vi "ExternalIN.vi"(0 "nDeviceNo":u32, 1 "Mode":u16(ring) items=["Get&Set", "Get", "Set"], 5 "nChildNo":u32, 9 "NewExternalInMode":u32[](array[numeric]), 11 "Error_In":T1) -> (3 "ExternalIn1ModeList":cluster{string, i32}[](array[cluster]), 4 "Error?":bool, 6 "ExternalIn1Mode":u32, 8 "ExternalIn2Mode":u32, 10 "ExternalIn3Mode":u32, 12 "ExternalIn2ModeList":cluster{string, i32}[](array[cluster]), 14 "ExternalIn3ModeList":cluster{string, i32}[](array[cluster]), 15 "Error_Out":T1)   [LabVIEW 2015]
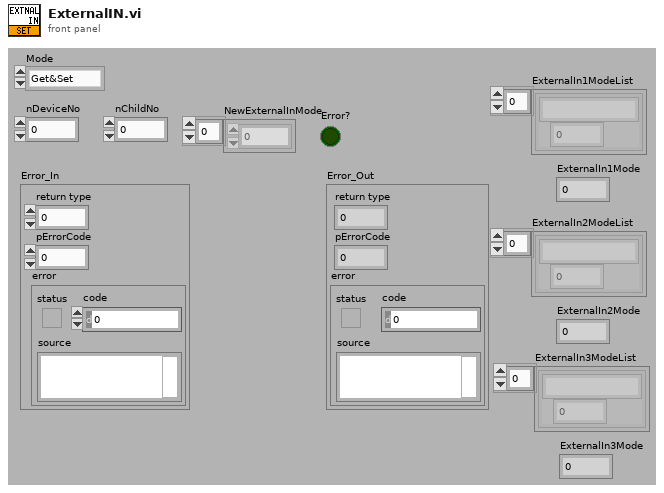
[diagram p1: front panel]
types:
  T1 = cluster{"return type":u32, "pErrorCode":u32, "error ":errorcluster}
  T2 = cluster{"ReturnValue":u32, "ErrorCode":u32, "error ":errorcluster}
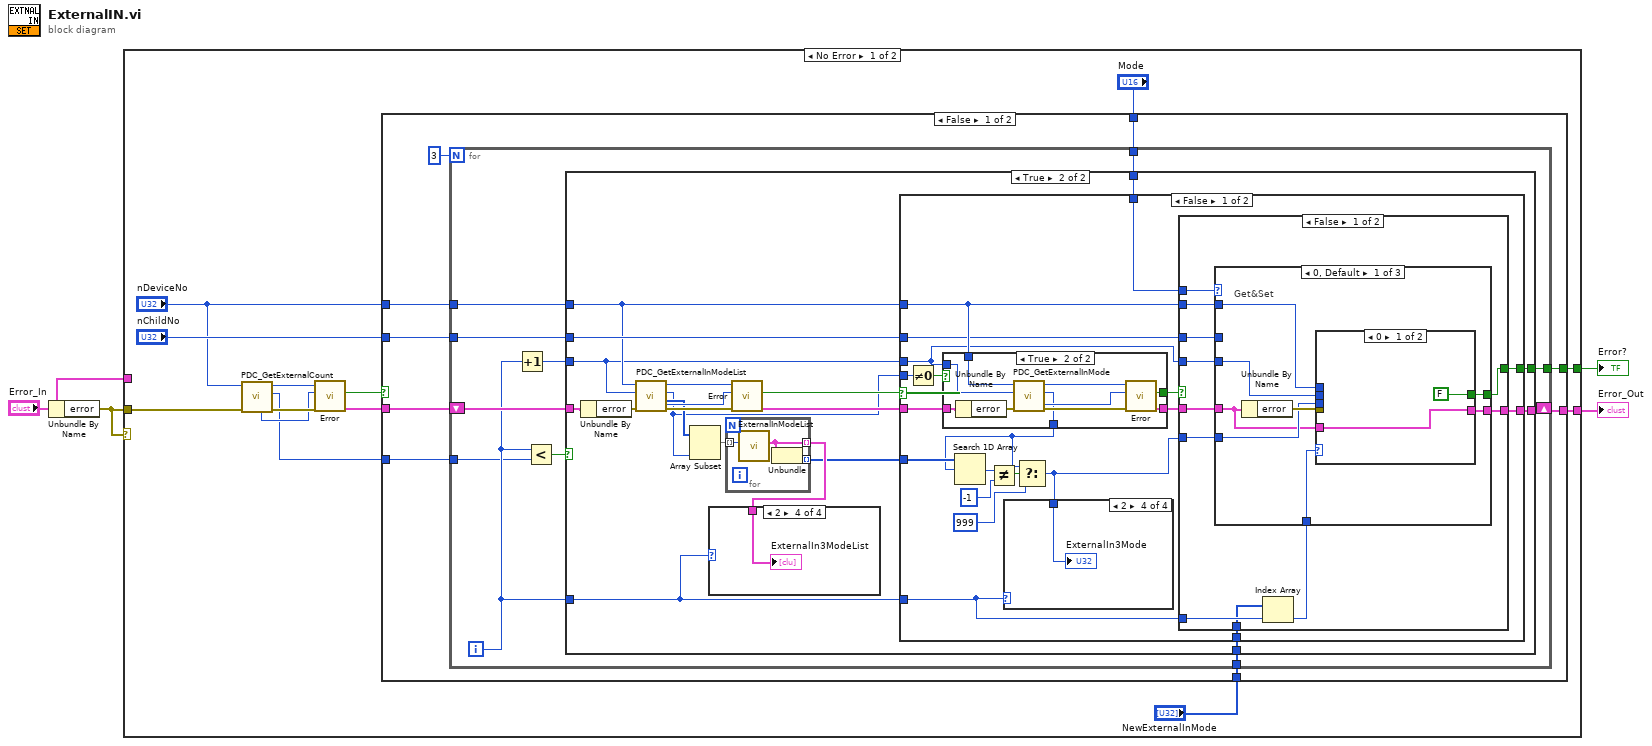
[diagram p0: block diagram]
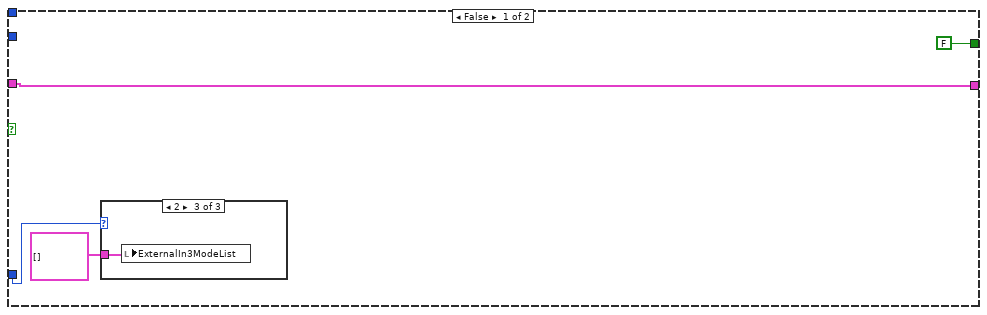
[diagram p2: hidden frame]
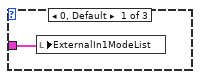
[diagram p3: hidden frame]
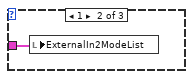
[diagram p4: hidden frame]
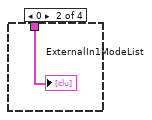
[diagram p6: hidden frame]
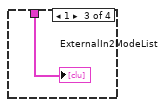
[diagram p7: hidden frame]
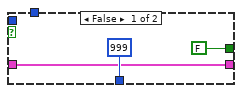
[diagram p8: hidden frame]
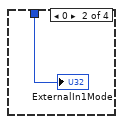
[diagram p10: hidden frame]
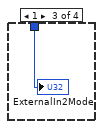
[diagram p11: hidden frame]
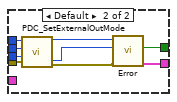
[diagram p12: hidden frame]
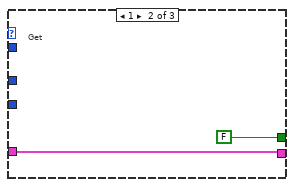
[diagram p13: hidden frame]
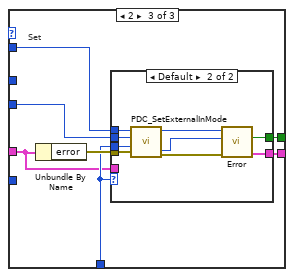
[diagram p14: hidden frame]
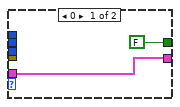
[diagram p15: hidden frame]
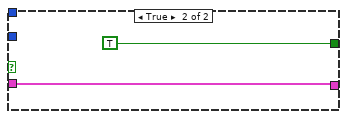
[diagram p16: hidden frame]
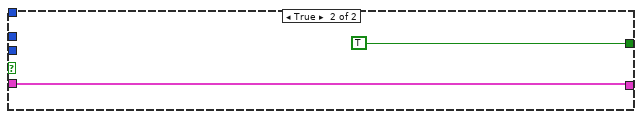
[diagram p17: hidden frame]
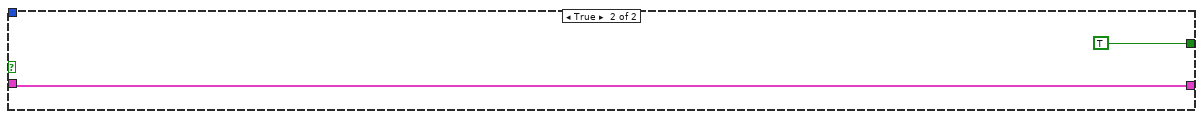
[diagram p18: hidden frame]
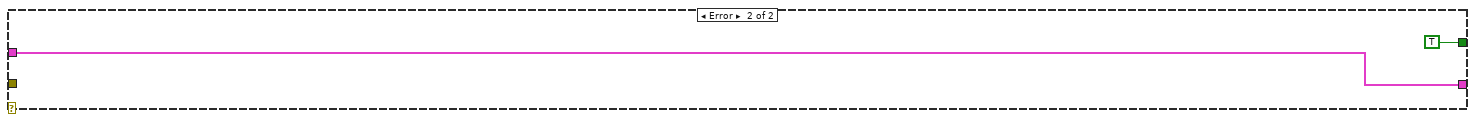
[diagram p19: hidden frame]
diagram:
  n1 = Unbundle By Name("Error_In") -> ("error"=w2:errorcluster)
  n2 = case shown="No Error" w2 {
    tunnel: [w17 w164] -> w4
    tunnel: [w16 TRUE ("Error?")] -> w3
    tunnel: w2 -> [w9 _]
    tunnel: "Error_In" -> [_ w164]
    frame No Error {
      n3 = call "PDC_GetExternalCount.vi"("error in (no error)"=w9, "DeviceNo"="nDeviceNo") -> ("error out"=w10:errorcluster, "In"=w5:u32, "ReturnValue"=w6:u32, "ErrorCode"=w7:u32)  [unwired: 6 out]
      n4 = call "Error.vi"("error in (no error)"=w10, "ErrorCode"=w7, "ReturnValue"=w6) -> ("Error_Out"=w12:T2, "Error?"=w13:bool)  [unwired: 7 out]
      n5 = case shown="False" w13 {
        tunnel: [w26 w161] -> w17
        tunnel: [w25 TRUE ("Error?")] -> w16
        tunnel: "nChildNo" -> [w24 _]
        tunnel: "nDeviceNo" -> [w23 _]
        tunnel: "Mode" -> [w22 _]
        tunnel: w12 -> [w21 w161]
        tunnel: "NewExternalInMode" -> [w20 _]
        tunnel: w5 -> [w18 _]
        frame False {
          n6 = for {
            N: 3 -> [_]
            tunnel: [w36] -> w25
            tunnel: w24 -> [w35]
            tunnel: w23 -> [w34]
            tunnel: w22 -> [w33]
            shift-right: [w37] -> w26
            shift-left: w21 -> [w32]
            tunnel: w20 -> [w31]
            tunnel: w18 -> [w27]
            i -> [w28]
            n7 = Increment(x=w28) -> (x+1=w30:i32)
            n8 = Less?(x=w28, y=w27) -> (x < y?=w29:bool)
            n9 = case shown="True" w29 {
              tunnel: [w41 w64] -> w37
              tunnel: [FALSE ("Error?") w63] -> w36
              tunnel: w35 -> [_ w62]
              tunnel: w34 -> [_ w55]
              tunnel: w33 -> [_ w53]
              tunnel: w32 -> [w41 w52]
              tunnel: w28 -> [w39 w50]
              tunnel: w30 -> [_ w49]
              tunnel: w31 -> [_ w48]
              frame False {
                n10 = case shown="2" w39 {
                  tunnel: cluster{string, i32}[] [] ("External\nGeneralOutModeList") -> [w42 w43 w44]
                  frame 0, Default {
                    n11 = local write "ExternalIn1ModeList"(w42) -> ()
                  }
                  frame 1 {
                    n12 = local write "ExternalIn2ModeList"(w43) -> ()
                  }
                  frame 2 {
                    n13 = local write "ExternalIn3ModeList"(w44) -> ()
                  }
                }
              }
              frame True {
                n14 = Unbundle By Name(w52) -> ("error"=w51:errorcluster)
                n15 = call "PDC_GetExternalInModeList.vi"("error in (no error)"=w51, "PortNo"=w49, "DeviceNo"=w55) -> ("error out"=w61:errorcluster, "List"=w57:u32[], "Size"=w45:u32, "ReturnValue"=w60:u32, "ErrorCode"=w59:u32)  [unwired: 4 out]
                n16 = Array Subset(array=w57, length=w45) -> (w58:u32[])  [unwired: 1 in]
                n17 = for {
                  tunnel: w58 -> [w160] mode=indexing
                  tunnel: [w159] -> w47 mode=indexing
                  tunnel: [w158] -> w46 mode=indexing
                  n18 = call "ExternalInModeList.vi"("List"=w160) -> ("GetLUTModeList"=w159:cluster{string, i32})  [unwired: 10 out]
                  n19 = Unbundle(w159) -> (w158:i32)  [unwired: 1 out]
                }
                n20 = case shown="2" w50 {
                  tunnel: w47 -> [_ w65 w66 w67]
                  frame Default {
                  }
                  frame 0 {
                    "ExternalIn1ModeList" <- w65
                  }
                  frame 1 {
                    "ExternalIn2ModeList" <- w66
                  }
                  frame 2 {
                    "ExternalIn3ModeList" <- w67
                  }
                }
                n21 = call "Error.vi"("error in (no error)"=w61, "ErrorCode"=w59, "ReturnValue"=w60) -> ("Error_Out"=w56:T2, "Error?"=w54:bool)  [unwired: 7 out]
                n22 = case shown="False" w54 {
                  tunnel: [w85 w157] -> w64
                  tunnel: [w84 TRUE ("Error?")] -> w63
                  tunnel: w56 -> [w83 w157]
                  tunnel: w55 -> [w82 _]
                  tunnel: w62 -> [w81 _]
                  tunnel: w49 -> [w70 _]
                  tunnel: w53 -> [w80 _]
                  tunnel: w50 -> [w79 _]
                  tunnel: w48 -> [w78 _]
                  tunnel: w46 -> [w77 _]
                  tunnel: w45 -> [w68 _]
                  frame False {
                    n23 = Not Equal To 0?(x=w68) -> (x != 0?=w69:bool)
                    n24 = case shown="True" w69 {
                      tunnel: [FALSE ("Error?") w97] -> w87
                      tunnel: [w89 w96] -> w86
                      tunnel: w83 -> [w89 w94]
                      tunnel: w82 -> [_ w93]
                      tunnel: w70 -> [_ w92]
                      tunnel: [u32 999 ("pMode") w91] -> w74
                      frame False {
                      }
                      frame True {
                        n25 = Unbundle By Name(w94) -> ("error"=w95:errorcluster)
                        n26 = call "PDC_GetExternalInMode.vi"("error in (no error)"=w95, "Port"=w92, "DeviceNo"=w93) -> ("error out"=w98:errorcluster, "Mode"=w91:u32, "ReturnValue"=w99:u32, "ErrorCode"=w100:u32)  [unwired: 5 out]
                        n27 = call "Error.vi"("error in (no error)"=w98, "ErrorCode"=w100, "ReturnValue"=w99) -> ("Error_Out"=w96:T2, "Error?"=w97:bool)  [unwired: 7 out]
                      }
                    }
                    n28 = Search 1D Array(1D array=w77, element=w74) -> (index of element=w76:i32)  [unwired: 1 out]
                    n29 = Not Equal?(x=w76, y=-1) -> (x != y?=w73:bool)
                    n30 = Select(t=w74, s=w73, f=u32 999 ("y")) -> (s? t:f=w72:u32)
                    n31 = case shown="2" w79 {
                      tunnel: w72 -> [_ w101 w102 w103]
                      frame Default {
                      }
                      frame 0 {
                        "ExternalIn1Mode" <- w101
                      }
                      frame 1 {
                        "ExternalIn2Mode" <- w102
                      }
                      frame 2 {
                        "ExternalIn3Mode" <- w103
                      }
                    }
                    n32 = case shown="False" w87 {
                      tunnel: w86 -> [w108 w155]
                      tunnel: [w114 w155] -> w85
                      tunnel: w82 -> [w111 _]
                      tunnel: w81 -> [w110 _]
                      tunnel: [w113 TRUE ("Error?")] -> w84
                      tunnel: w80 -> [w112 _]
                      tunnel: w72 -> [w109 _]
                      tunnel: w70 -> [w107 _]
                      tunnel: w79 -> [w106 _]
                      tunnel: w78 -> [w105 _]
                      frame False {
                        n33 = Index Array(array=w105, index=w106) -> (element=w104:u32)
                        n34 = case shown="0, Default" w112 {
                          tunnel: w108 -> [w115 w135 w136]
                          tunnel: [w121 w135 w141] -> w114
                          tunnel: w111 -> [w120 _ w140]
                          tunnel: w110 -> [_ _ _]
                          tunnel: [w119 FALSE ("Error?") w139] -> w113
                          tunnel: w109 -> [w118 _ _]
                          tunnel: w107 -> [w117 _ w138]
                          tunnel: w104 -> [w116 _ w137]
                          frame 0, Default {
                            # "Get&Set"
                            n35 = Unbundle By Name(w115) -> ("error"=w122:errorcluster)
                            n36 = case shown="0" w116 {
                              tunnel: w122 -> [_ w133]
                              tunnel: [w123 w129] -> w121
                              tunnel: w120 -> [_ w128]
                              tunnel: [FALSE ("Error?") w127] -> w119
                              tunnel: w118 -> [_ w126]
                              tunnel: w117 -> [_ w125]
                              tunnel: w115 -> [w123 _]
                              frame 0 {
                              }
                              frame Default {
                                n37 = call "PDC_SetExternalOutMode.vi"("error in (no error)"=w133, "Mode"=w126, "Port"=w125, "DeviceNo"=w128) -> ("error out"=w130:errorcluster, "ReturnValue"=w132:u32, "ErrorCode"=w131:u32)  [unwired: 5 out]
                                n38 = call "Error.vi"("error in (no error)"=w130, "ErrorCode"=w131, "ReturnValue"=w132) -> ("Error_Out"=w129:T2, "Error?"=w127:bool)  [unwired: 7 out]
                              }
                            }
                          }
                          frame 1 {
                            # "Get"
                          }
                          frame 2 {
                            # "Set"
                            n39 = Unbundle By Name(w136) -> ("error"=w142:errorcluster)
                            n40 = case shown="Default" w137 {
                              tunnel: w142 -> [_ w153]
                              tunnel: [w143 w149] -> w141
                              tunnel: w140 -> [_ w148]
                              tunnel: [FALSE ("Error?") w147] -> w139
                              tunnel: w138 -> [_ w146]
                              tunnel: w137 -> [_ w145]
                              tunnel: w136 -> [w143 _]
                              frame 0 {
                              }
                              frame Default {
                                n41 = call "PDC_SetExternalInMode.vi"("error in (no error)"=w153, "Mode"=w145, "Port"=w146, "DeviceNo"=w148) -> ("error out"=w150:errorcluster, "ReturnValue"=w152:u32, "ErrorCode"=w151:u32)  [unwired: 5 out]
                                n42 = call "Error.vi"("error in (no error)"=w150, "ErrorCode"=w151, "ReturnValue"=w152) -> ("Error_Out"=w149:T2, "Error?"=w147:bool)  [unwired: 7 out]
                              }
                            }
                          }
                        }
                      }
                      frame True {
                      }
                    }
                  }
                  frame True {
                  }
                }
              }
            }
          }
        }
        frame True {
        }
      }
    }
    frame Error {
    }
  }
  "Error_Out" <- w4
  "Error?" <- w3
